vi "ConfigWfrm.vi"(5 "Offset":dbl, 7 "Gain":dbl, 8 "error in (no error)":errorcluster, 9 "Handle":string, 10 "ChannelName":string, 11 "ArbitraryFunction in":refnum<class "ArbitraryFunction.lvclass">) -> (0 "error out":errorcluster, 3 "ArbitraryFunction out":refnum<class "ArbitraryFunction.lvclass">)   [LabVIEW 2014, in "Functions.lvlib" / "ArbitraryFunction.lvclass"]
uses:
  ArbitraryFunction.lvclass
  ArbitraryFunction.lvclass/ArbitraryFunction.ctl
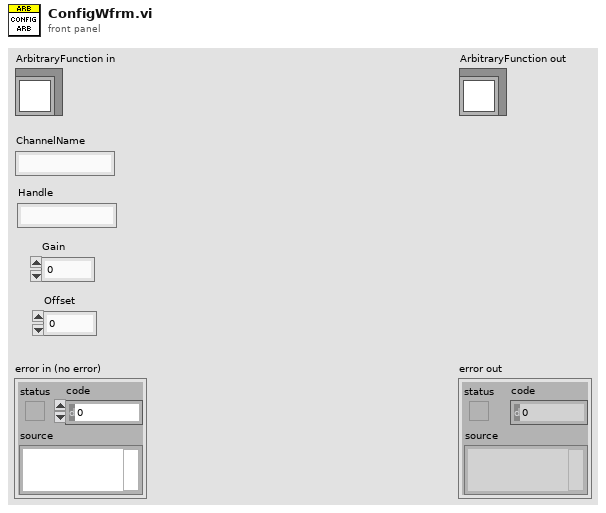
[diagram p1: front panel]
types:
  T1 = typedef "Functions.lvlib/ArbitraryFunction.lvclass/Arbitrary.ctl" = cluster{"Handle":string, "Size":i32, "Gain":dbl, "Offset":dbl, "Waveform":waveform(dbl)}
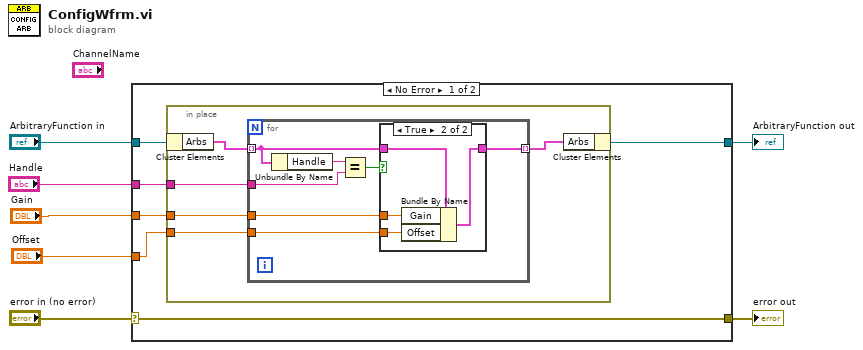
[diagram p0: block diagram]
diagram:
  n1 = case shown="No Error" "error in (no error)" {
    selector: "error in (no error)" -> [w13 w32]
    tunnel: [w13 w32] -> w6
    tunnel: [w8 w31] -> w4
    tunnel: "ArbitraryFunction in" -> [w12 w31]
    tunnel: "Handle" -> [w11 _]
    tunnel: "Gain" -> [w10 _]
    tunnel: "Offset" -> [w9 _]
    frame No Error {
      n2 = in-place {
        in-place-border: w11 -> [w17]
        in-place-border: w10 -> [w16]
        in-place-border: w9 -> [w15]
        n3 = in-place-cluster #1(w12) -> ("Arbs"=w18:T1[])
        n4 = for {
          tunnel: w18 -> [w23] mode=indexing
          tunnel: w17 -> [w24]
          tunnel: w16 -> [w21]
          tunnel: w15 -> [w20]
          tunnel: [w19] -> w14 mode=indexing
          n5 = Unbundle By Name(w23) -> ("Handle"=w25:string)
          n6 = Equal?(x=w25, y=w24) -> (x = y?=w22:bool)
          n7 = case shown="True" w22 {
            tunnel: w23 -> [w26 w30]
            tunnel: w21 -> [_ w29]
            tunnel: w20 -> [_ w28]
            tunnel: [w26 w27] -> w19
            frame False {
            }
            frame True {
              n8 = Bundle By Name(cluster=w30, "Gain"=w29, "Offset"=w28) -> (w27:T1)
            }
          }
        }
        n9 = in-place-cluster #1("Arbs"=w14) -> (w8:refnum<class "ArbitraryFunction.lvclass">)
      }
    }
    frame Error {
    }
  }
  "error out" <- w6
  "ArbitraryFunction out" <- w4
